vi "DAQ_Manager.TestLauncher.vi"() -> ()   [LabVIEW 2019, in "DAQ_Manager.lvclass"]
uses:
  DAQ_Manager.lvclass
  <vilib>/JKI/JKI SMO/SMO/SMO.lvclass
  <vilib>/JKI/JKI SMO/SMO/Typedefs/SMOState --Enum.ctl
  C:/Program Files (x86)/National Instruments/LabVIEW 2016/vi.lib/JKI/JKI SMO/SMO/SMO.lvclass
  Typedefs/PrivateEvents--DAQ_Manager.setDAQConfig.ctl
  DAQmx.AO/Typedefs/DAQmx.AO_Config.ctl
  DAQmx.AI/Typedefs/DAQmx.AI_Config.ctl
  DAQmx.AI/Typedefs/AI.Coupling-enum.ctl
  DAQmx.AI/Typedefs/AI.Terminal-enum.ctl
  DAQmx.AO/Typedefs/AO.Terminal-enum.ctl
panel:
  in  "DAQ_Manager.setDAQConfig":T1={"DAQ.Config (AI)"=[{"Channels"="PXI1Slot2/ai0:1", "DAQ_Type"=enum."AI", "minimum value"=-0.3, "maximum value"=0.3, "DAQ_SamplingInfo"={"Fs"=10000.0, "#s"=1000}, "DAQ_SamplingMode"=enum."Continuous"}, {"Channels"="PXI1Slot3/ai0:1", "DAQ_Type"=enum."AI", "minimum value"=-0.3, "maximum value"=0.3, "DAQ_SamplingInfo"={"Fs"=10000.0, "#s"=1000}, "DAQ_SamplingMode"=enum."Continuous"}, {"Channels"="PXI1Slot4/ai0:1", "DAQ_Type"=enum."AI", "minimum value"=-0.3, "maximum value"=0.3, "DAQ_SamplingInfo"={"Fs"=10000.0, "#s"=1000}, "DAQ_SamplingMode"=enum."Continuous"}], "DAQmx.AI.config"=[{"AI.Coupling"=10045, "input terminal configuration "=-1}, {"AI.Coupling"=10045, "input terminal configuration "=-1}, {"AI.Coupling"=10045, "input terminal configuration "=-1}], "DAQ.Config (AO)"=[{"Channels"="PXI1Slot2/ao0:1", "DAQ_Type"=enum."AO", "minimum value"=-0.1, "maximum value"=0.1, "DAQ_SamplingInfo"={"Fs"=10000.0, "#s"=1000}, "DAQ_SamplingMode"=enum."Continuous"}, {"Channels"="PXI1Slot3/ao0:1", "DAQ_Type"=enum."AO", "minimum value"=-0.1, "maximum value"=0.1, "DAQ_SamplingInfo"={"Fs"=10000.0, "#s"=1000}, "DAQ_SamplingMode"=enum."Continuous"}, {"Channels"="PXI1Slot4/ao0:1", "DAQ_Type"=enum."AO", "minimum value"=-0.1, "maximum value"=0.1, "DAQ_SamplingInfo"={"Fs"=10000.0, "#s"=1000}, "DAQ_SamplingMode"=enum."Continuous"}], "DAQmx.AO.config"=[{"output terminal configuration"=-1}, {"output terminal configuration"=-1}, {"output terminal configuration"=-1}]} {"DAQmx.AI.config"."input terminal configuration" items=["default"=-1, "RSE"=10083, "NRSE"=10078, "Differential"=10106, "Pseudodifferential"=12529]; "DAQmx.AI.config"."AI.Coupling" items=["AC"=10045, "DC"=10050, "GND"=10066]; "DAQmx.AO.config"."output terminal configuration" items=["Default"=-1, "RSE"=10083, "Differential"=10106, "Pseudodifferential"=12529]}
  in  "setDAQConfig":bool
  out "getWaveforms":waveform(dbl)[](graph)=[{"t0"=timestamp(3592827387.4344635 s since 1904-01-01), "dt"=9.99999999114152e-05, "Y"=array[1000 elements], "attributes"=variant("NI_ChannelName"=variant(string "PXI1Slot2/ai0"), "NI_UnitDescription"=variant(string "Volts"))}, {"t0"=timestamp(3592827387.4344635 s since 1904-01-01), "dt"=9.99999999114152e-05, "Y"=array[1000 elements], "attributes"=variant("NI_ChannelName"=variant(string "PXI1Slot2/ai1"), "NI_UnitDescription"=variant(string "Volts"))}, {"t0"=timestamp(3592827387.4008803 s since 1904-01-01), "dt"=9.99999999114152e-05, "Y"=array[1000 elements], "attributes"=variant("NI_ChannelName"=variant(string "PXI1Slot3/ai0"), "NI_UnitDescription"=variant(string "Volts"))}, {"t0"=timestamp(3592827387.4008803 s since 1904-01-01), "dt"=9.99999999114152e-05, "Y"=array[1000 elements], "attributes"=variant("NI_ChannelName"=variant(string "PXI1Slot3/ai1"), "NI_UnitDescription"=variant(string "Volts"))}, {"t0"=timestamp(3592827387.472322 s since 1904-01-01), "dt"=9.99999999114152e-05, "Y"=array[1000 elements], "attributes"=variant("NI_ChannelName"=variant(string "PXI1Slot4/ai0"), "NI_UnitDescription"=variant(string "Volts"))}]
  out "SMO State":T7=enum."Stopped"
  out "error out":errorcluster
  in  "Stop":bool
  # "DAQ Manager SMO Test Launcher"
  # "For instructions on how to use the JKI State Machine Objects, examples and video tutorials, visit:\nhttp://jki.net/state-machine-objects/\n\nJKI State Machine Objects™\nhttp://jki.net/state-machine-objects/\nCopyright (C) 2005-2015, JKI <info@jki.net>\nALL RIGHTS RESERVED"
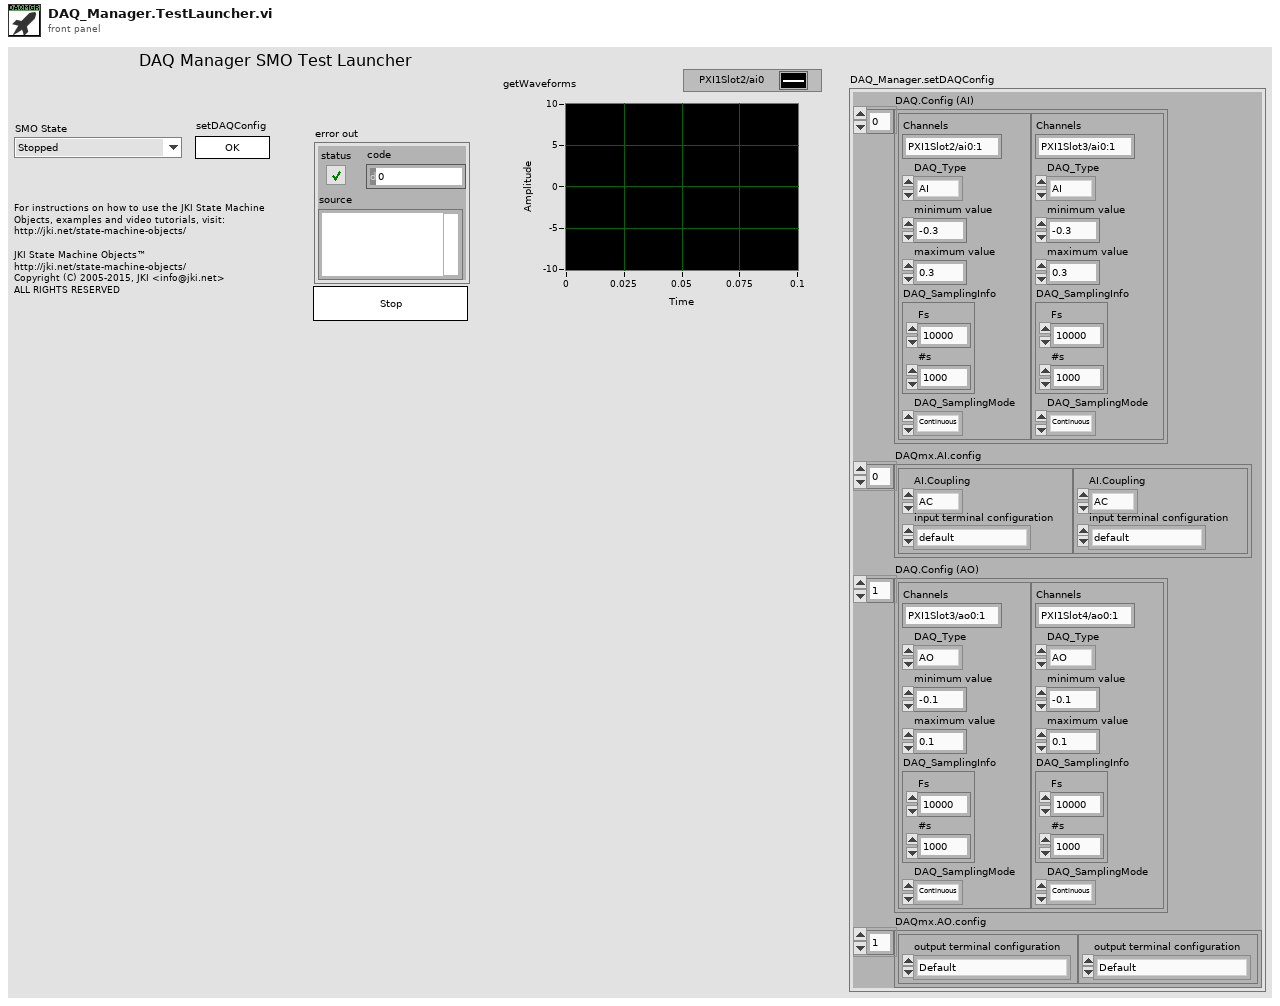
[diagram p1: front panel]
types:
  T1 = typedef "DAQ_Manager.lvclass/PrivateEvents--DAQ_Manager.setDAQConfig.ctl" = cluster{"DAQ.Config (AI)":cluster{"Channels":string, "DAQ_Type":enum16{"AI", "AO"}, "minimum value":dbl, "maximum value":dbl, "DAQ_SamplingInfo":cluster{"Fs":dbl, "#s":i32}, "DAQ_SamplingMode":enum16{"Continuous", "Finite"}}[], "DAQmx.AI.config":T2[], "DAQ.Config (AO)":cluster{"Channels":string, "DAQ_Type":enum16{"AI", "AO"}, "minimum value":dbl, "maximum value":dbl, "DAQ_SamplingInfo":cluster{"Fs":dbl, "#s":i32}, "DAQ_SamplingMode":enum16{"Continuous", "Finite"}}[], "DAQmx.AO.config":T5[]}
  T2 = typedef "DAQmx.AI.lvclass/DAQmx.AI_Config.ctl" = cluster{"AI.Coupling":T3, "input terminal configuration ":T4}
  T3 = typedef "DAQmx.AI.lvclass/AI.Coupling-enum.ctl" = i32
  T4 = typedef "DAQmx.AI.lvclass/AI.Terminal-enum.ctl" = i32
  T5 = typedef "DAQmx.AO.lvclass/DAQmx.AO_Config.ctl" = cluster{"output terminal configuration":T6}
  T6 = typedef "DAQmx.AO.lvclass/AO.Terminal-enum.ctl" = i32
  T7 = typedef "SMO.lvclass/SMOState --Enum.ctl" = enum16{"unknown", "Created", "Started", "Stopped"}
  T8 = typedef "SMO.lvclass/Public Events.ctl" = cluster{"Error":refnum<user-event>, "State":refnum<user-event>, "Reserve State":refnum<user-event>}
  T9 = typedef "DAQ_Manager.lvclass/PublicEvents--Cluster.ctl" = cluster{"getWaveform":refnum<user-event>}
  T10 = cluster{"Event Registration Refnum":refnum<event-registration>}
  T11 = typedef "DAQ_Manager.lvclass/PublicEvents--DAQ_Manager.getWaveform.ctl" = waveform(dbl)[]
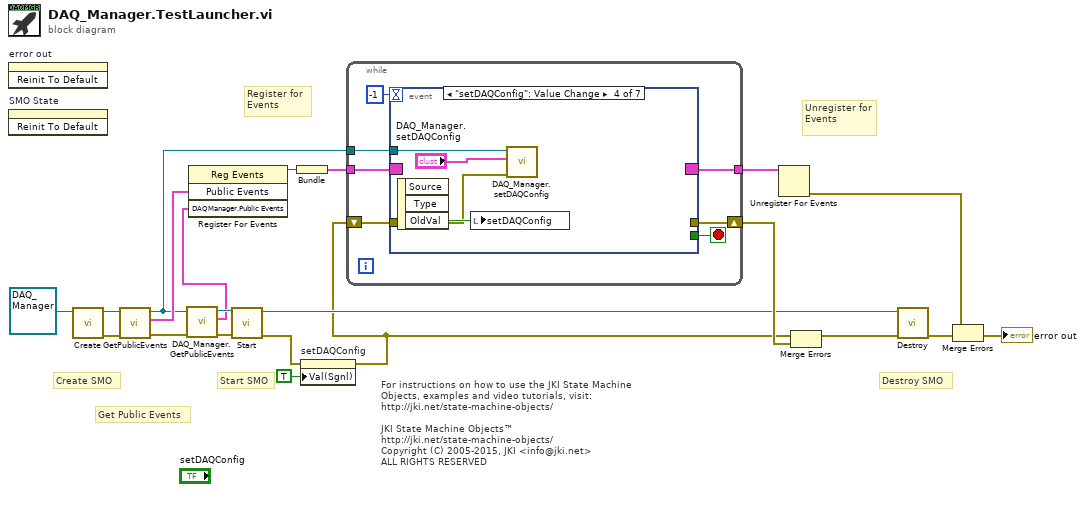
[diagram p0: block diagram]
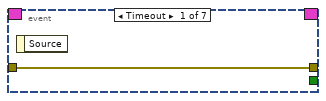
[diagram p2: hidden frame]
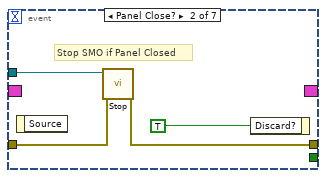
[diagram p3: hidden frame]
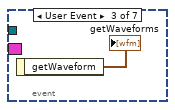
[diagram p4: hidden frame]
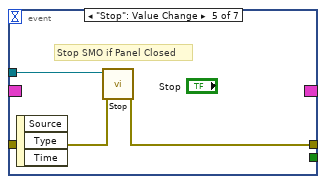
[diagram p5: hidden frame]
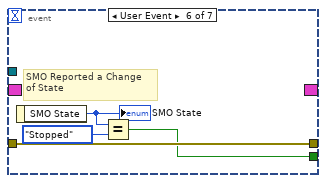
[diagram p6: hidden frame]
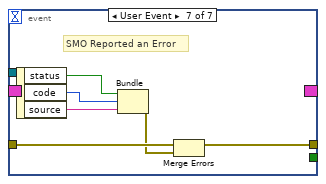
[diagram p7: hidden frame]
diagram:
  # "For instructions on how to use the JKI State Machine Objects, examples and video tutorials, visit:\nhttp://jki.net/state-machine-objects/\n\nJKI State Machine Objects™\nhttp://jki.net/state-machine-objects/\nCopyright (C) 2005-2015, JKI <info@jki.net>\nALL RIGHTS RESERVED"
  # "Get Public Events"
  # "Start SMO"
  # "Destroy SMO"
  # "Create SMO"
  # "Unregister for Events"
  # "Register for Events"
  n1 = invoke on="error out" class="Clust (strict)" method="Reinit To Default"() -> ()  [unwired: 3 in, 3 out]
  n2 = invoke on="SMO State" class="Enum (strict)" method="Reinit To Default"() -> ()  [unwired: 3 in, 3 out]
  n3 = call <vilib>:"Create.vi"("SMO"=refnum<class "DAQ_Manager.lvclass"> refnum ("SMO.Template.lvclass")) -> ("error out"=w12:errorcluster, "SMO out"=w13:refnum<class "DAQ_Manager.lvclass">)  [unwired: 8 in, 1 out]
  n4 = call <vilib>:"GetPublicEvents.vi"("error in (no error)"=w12, "SMO"=w13) -> ("error out"=w9:errorcluster, "Public Events"=w11:T8, "SMO out"=w8:refnum<class "DAQ_Manager.lvclass">)  [unwired: 7 in]
  n5 = call "DAQ_Manager.GetPublicEvents.vi"("error in (no error)"=w9, "DAQ_Manager"=w8) -> ("error out"=w5:errorcluster, "DAQManager.Public Events"=w6:T9, "DAQ_Manager out"=w7:refnum<class "DAQ_Manager.lvclass">)  [unwired: 7 in]
  n6 = register-events(w11, w6) -> (reference out=w10:refnum<event-registration>)  [unwired: 2 in, 1 out]
  n7 = call <vilib>:"Start.vi"("error in (no error)"=w5, "SMO"=w7) -> ("error out"=w3:errorcluster, "SMO out"=w4:refnum<class "DAQ_Manager.lvclass">)  [unwired: 8 in]
  n8 = Bundle("Event Registration Refnum"=w10) -> (w20:T10)  [unwired: 1 in]
  n9 = property on="setDAQConfig" class="Bool (strict)"(error in=w3, "Val(Sgnl)"=TRUE ("Value (Signaling)")) -> (error out=w2:errorcluster)  [unwired: 1 in, 1 out]
  n10 = while {
    shift-right: [w27] -> w19
    shift-left: w2 -> [w26]
    tunnel: w20 -> [w25]
    tunnel: [w24] -> w21
    tunnel: w8 -> [w23]
    stop <- w28 stop-if-true
    n11 = event shown="[3] \"setDAQConfig\": Value Change" {
      selector: w25 -> [_ _ _ _ _ _ _]
      dyn-events: [_ _ _ _ _ _ _] -> w24
      timeout: -1 -> [_ _ _ _ _ _ _]
      tunnel: [_ _ _ _ _ w43 _] -> w28
      tunnel: w23 -> [_ w33 _ w35 w41 _ _]
      tunnel: [w29 w32 _ _ w40 w45 w49] -> w27
      tunnel: w26 -> [w29 w31 _ w37 w39 w45 w47]
      event Timeout {
        n12 = event-data() -> ()  [unwired: 1 in, 1 out]
      }
      event Panel Close? {
        # "Stop SMO if Panel Closed"
        n13 = event-data() -> ()  [unwired: 1 in, 1 out]
        n14 = call <vilib>:"Stop.vi"("error in (no error)"=w31, "SMO"=w33) -> ("error out"=w32:errorcluster)  [unwired: 8 in, 1 out]
        n15 = event-data("Discard?"=TRUE ("OK")) -> ()  [unwired: 1 in, 1 out]
      }
      event User Event {
        n16 = event-data() -> ("getWaveform"=→"getWaveforms":T11)  [unwired: 1 in]
      }
      event "setDAQConfig": Value Change {
        n17 = event-data() -> ("OldVal"=w38:bool)  [unwired: 1 in, 2 out]
        n18 = local write "setDAQConfig"(w38) -> ()
        n19 = call "DAQ_Manager.setDAQConfig.vi"("error in (no error)"=w37, "DAQ_Manager.setDAQConfig"="DAQ_Manager.setDAQConfig", "DAQ_Manager"=w35) -> ()  [unwired: 7 in, 2 out]
      }
      event "Stop": Value Change {
        # "Stop SMO if Panel Closed"
        n20 = event-data() -> ()  [unwired: 1 in, 3 out]
        n21 = call <vilib>:"Stop.vi"("error in (no error)"=w39, "SMO"=w41) -> ("error out"=w40:errorcluster)  [unwired: 8 in, 1 out]
      }
      event User Event {
        # "SMO Reported a Change\nof State"
        n22 = event-data() -> ("SMO State"=w42:T7)  [unwired: 1 in]
        "SMO State" <- w42
        n23 = Equal?(x=w42, y=SMOState_--Enum."Stopped") -> (x = y?=w43:bool)
      }
      event User Event {
        # "SMO Reported an Error"
        n24 = event-data() -> ("status"=w48:bool, "code"=w51:i32, "source"=w50:string)  [unwired: 1 in]
        n25 = Bundle("status"=w48, "code"=w51, "source"=w50) -> (w46:errorcluster)  [unwired: 1 in]
        n26 = Merge Errors(w47, w46) -> (w49:errorcluster)
      }
    }
  }
  n27 = Unregister For Events(event registration refnum=w21) -> (error out=w18:errorcluster)  [unwired: 1 in]
  n28 = Merge Errors(w2, w19) -> (w14:errorcluster)
  n29 = call <vilib>:"Destroy.vi"("error in (no error)"=w14, "SMO"=w4) -> ("error out"=w16:errorcluster)  [unwired: 9 in]
  n30 = Merge Errors(w18, w16) -> (→"error out":errorcluster)
